vi "To String.vi"(8 "error in (no error)":errorcluster, 10 "Parameters":variant, 11 "Data2D in":refnum<class "Data2D.lvclass">) -> (0 "error out":errorcluster, 2 "String":string, 3 "Data2D out":refnum<class "Data2D.lvclass">)   [LabVIEW 2014, in "Data2D.lvclass"]
uses:
  Data2D.lvclass
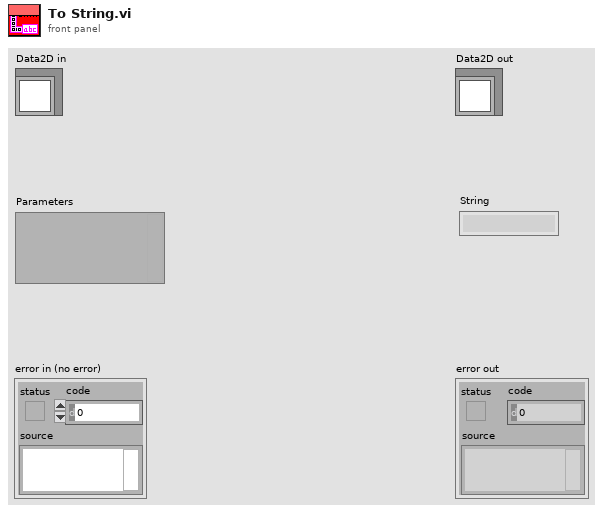
[diagram p1: front panel]
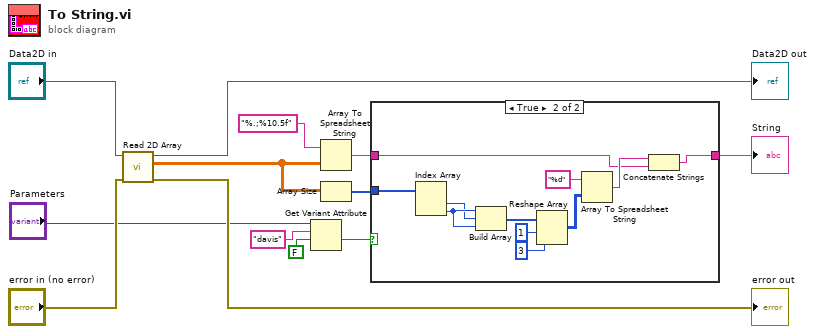
[diagram p0: block diagram]
diagram:
  n1 = call "Read 2D Array.vi"("error in (no error)"="error in (no error)", "Data2D in"="Data2D in") -> ("error out"=→"error out":errorcluster, "2D Array"=w2:dbl[][], "Data2D out"=→"Data2D out":refnum<class "Data2D.lvclass">)  [unwired: 7 in]
  n2 = Get Variant Attribute(Variant="Parameters", name="davis", default value (empty Variant)=FALSE) -> (value=w5:bool)  [unwired: 1 in, 3 out]
  n3 = Array To Spreadsheet String(array=w2, 3:"%.;%10.5f" ("format string")) -> (spreadsheet string=w4:string)  [unwired: 1 in]
  n4 = Array Size(array=w2) -> (size(s)=w1:i32[])
  n5 = case shown="True" w5 {
    tunnel: w4 -> [w14 w16]
    tunnel: [w14 w15] -> w3
    tunnel: w1 -> [_ w24]
    frame False {
    }
    frame True {
      n6 = Index Array(array=w24) -> (element #1=w22:i32, element #2=w23:i32)  [unwired: 2 in]
      n7 = Build Array(w23, w22, w23) -> (w21:i32[])
      n8 = Reshape Array(w21, 1 ("dimension size"), 3 ("dimension size")) -> (w18:i32[][])
      n9 = Array To Spreadsheet String(array=w18, 3:"%d" ("format string")) -> (spreadsheet string=w17:string)  [unwired: 1 in]
      n10 = Concatenate Strings(w17, w16) -> (w15:string)
    }
  }
  "String" <- w3
